vi "SiCenterFinder4Fids.vi"(0 "Operation":enum16{"Manual", "Automatic"}(ring)=enum."Automatic", 1 "Zone":enum16{"ZoneA", "ZoneB", "ZoneC", "ZoneD"}(ring), 2 "Autofocus":T2={"Enable"=TRUE, "InitialStepSize"=0.05, "Tolerance"=0.02, "Abort"=FALSE} {"Tolerance" format="%#_13g"}, 5 "Component":enum16{"Si", "SiOnBP"}(ring), 7 "VisibilityInCamera":enum16{"JoyStick", "AllVisible"}(ring)=enum."AllVisible", 11 "error in (no error)":errorcluster, 12 "Position":enum16{"1", "2"}(ring), 14 "SaveImagesLog":bool) -> (4 "Output XYZU":string, 6 "Image":T4(plugin-control), 8 "Image 2":T4[](array[plugin-control]) caption="AllImages", 15 "error out":errorcluster)   [LabVIEW 2021]
uses:
  <vilib>/userDefined/High Color/IMAQdx.ctl
  <vilib>/Analysis/coordinate.llb/2D Cartesian Coordinate Rotation (Scalar).vi
  <vilib>/Analysis/baseanly.llb/Mean (DBL).vi
  include/GlobalVariables.vi
  <vilib>/Analysis/NI_AALPro.lvlib
  <vilib>/Analysis/NI_AALBase.lvlib
  <vilib>/vision/driver/NI_Vision_Acquisition_Software.lvlib
panel:
  out "JoyStickStatus":bool
  out "Angle12":dbl
  out "Angle34":dbl
  in  "Camera":T1="cam1"
  in  "MatchParameters":T3={"Number of Matches Requested"=1, "Minimum Match Score"=700.0, "Angle Ranges"=[{"Start Angle"=0.0, "End Angle"=0.0}]}
  out "OutputFile":string
  out "spreadsheet string 2":string
  out "spreadsheet string":string
  in  "ModuleName":string="T1"
  out "SyringeY":dbl format="%#_7g"
  out "SyringeX":dbl format="%#_7g"
  in  "CamToSyringeYoffset":dbl=126.651
  in  "CamToSyringeXoffset":dbl=167.702
  out "FileUsedForFiducials":string
  out "UsedCoordinates":string
  out "CameraGcode":string
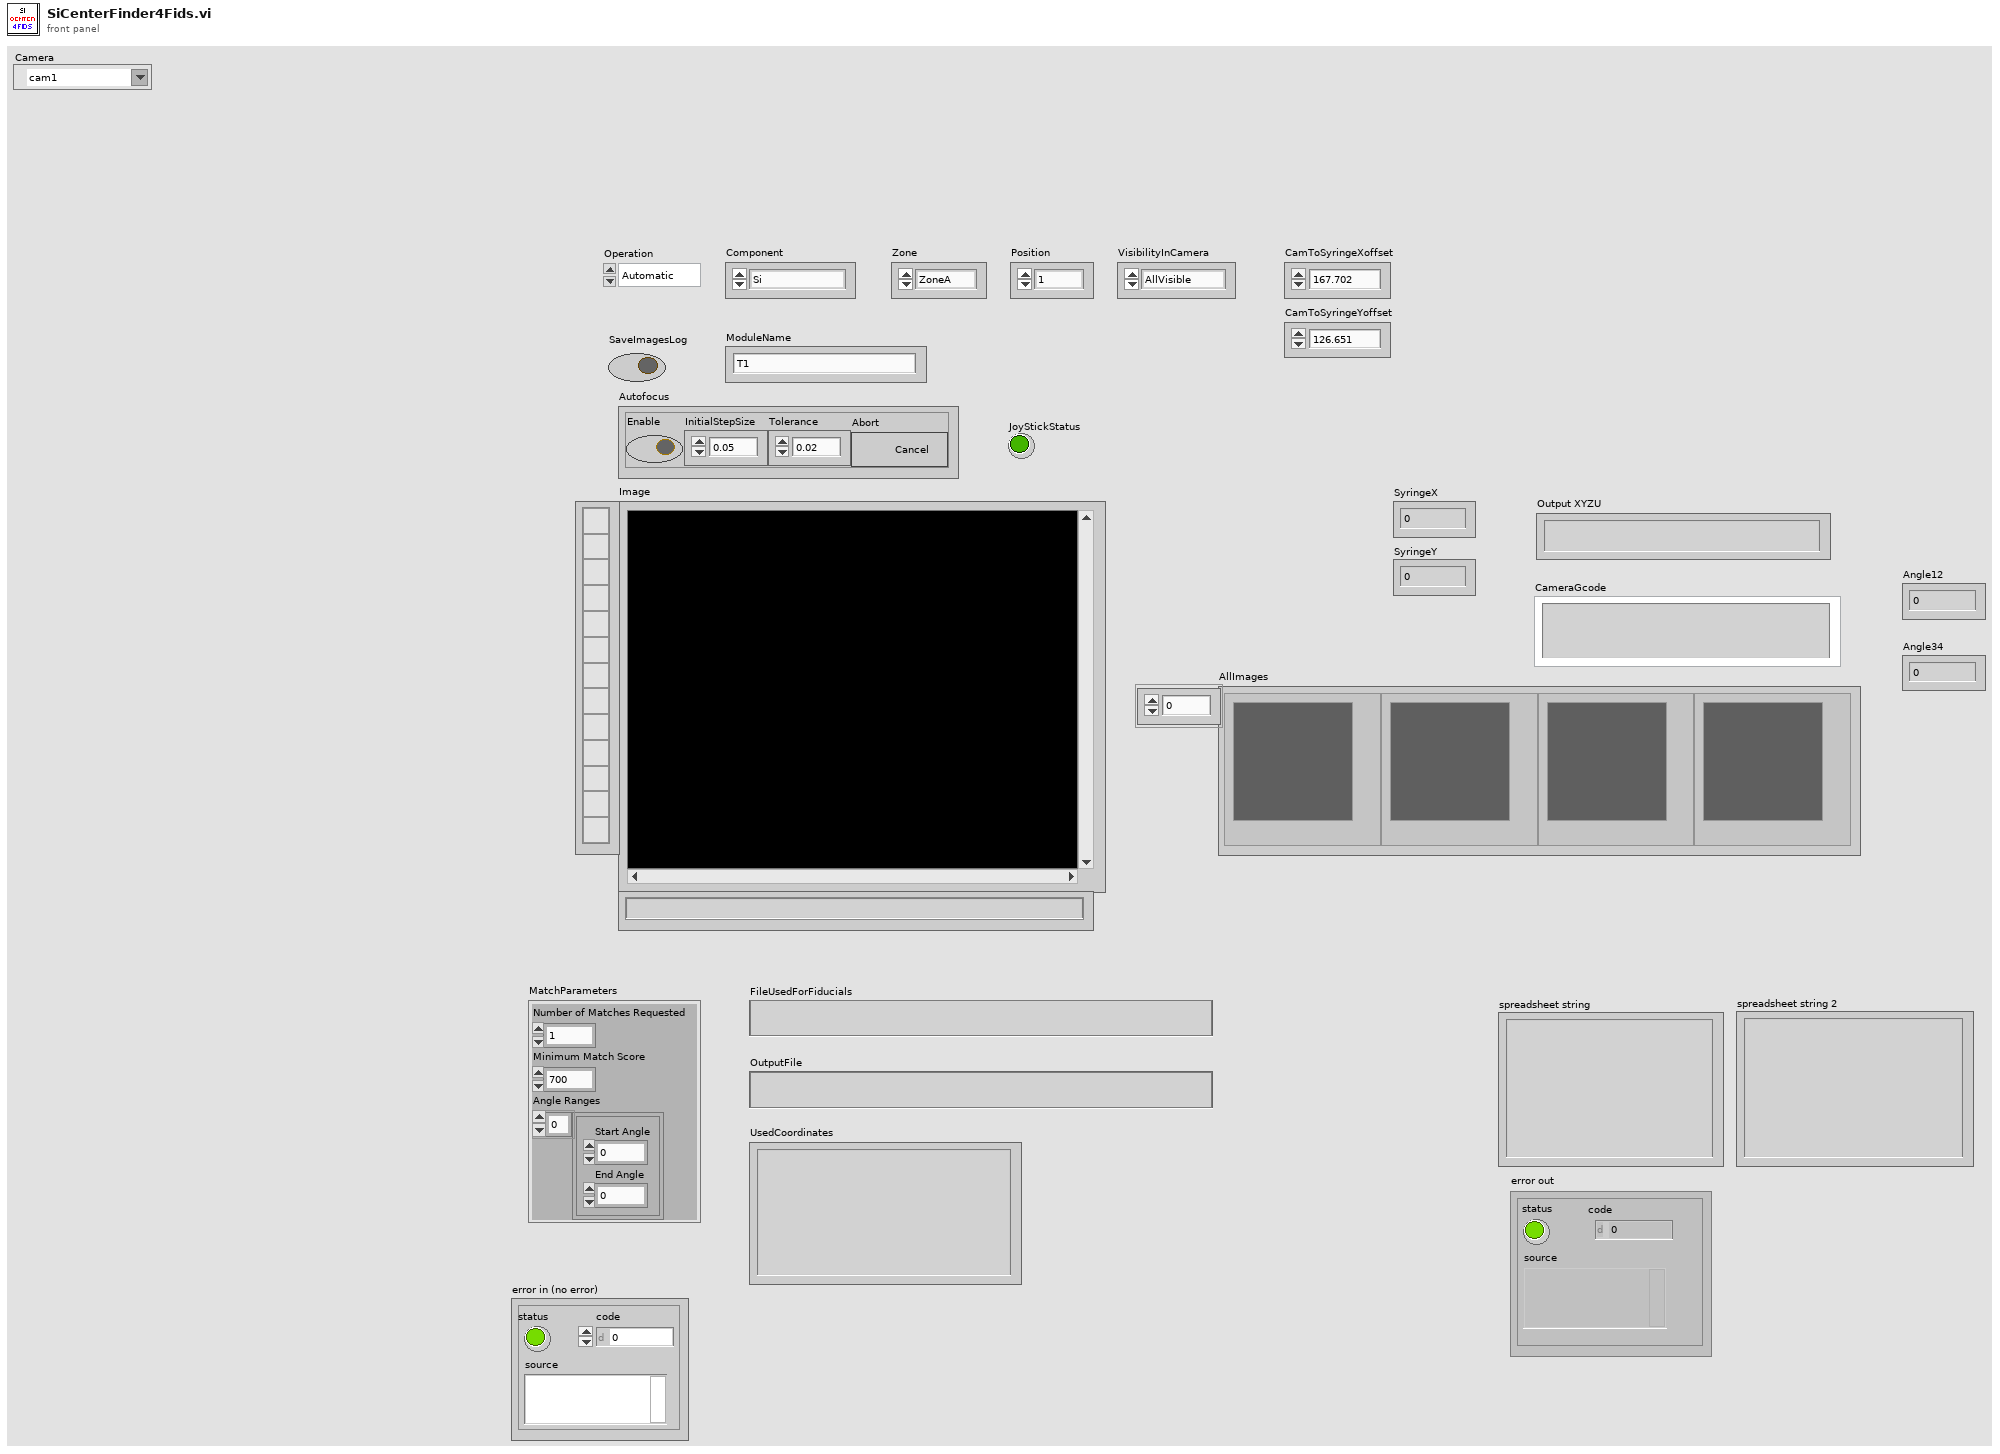
[diagram p1: front panel]
types:
  T1 = typedef "IMAQdx.ctl" = refnum<k21>
  T2 = cluster{"Enable":bool, "InitialStepSize":dbl, "Tolerance":dbl, "Abort":bool}
  T3 = cluster{"Number of Matches Requested":i32, "Minimum Match Score":sgl, "Angle Ranges":cluster{"Start Angle":sgl, "End Angle":sgl}[]}
  T4 = typedef "IMAQ Image.ctl" = refnum<image>
  T5 = typedef "Image Type" = u32
  T6 = typedef "IMAQ Point" = cluster{"X":sgl, "Y":sgl}
  T7 = enum16{"Left Button", "Center Button", "Right Button", "Window Close"}
  T8 = enum16{"open", "replace", "create", "open or create", "replace or create", "replace or create with confirmation"}
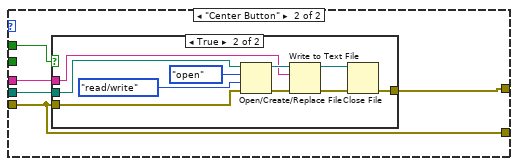
[diagram p5: hidden frame]
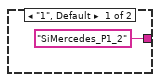
[diagram p7: hidden frame]
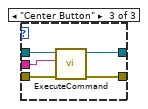
[diagram p10: hidden frame]
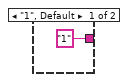
[diagram p11: hidden frame]
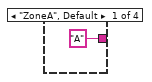
[diagram p12: hidden frame]
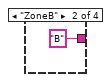
[diagram p13: hidden frame]
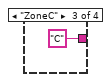
[diagram p14: hidden frame]
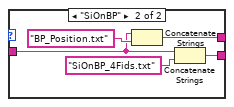
[diagram p15: hidden frame]
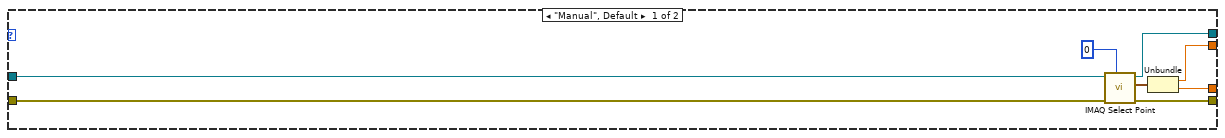
[diagram p16: hidden frame]
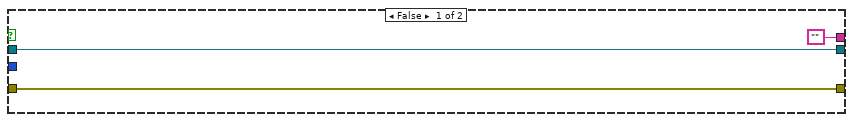
[diagram p18: hidden frame]
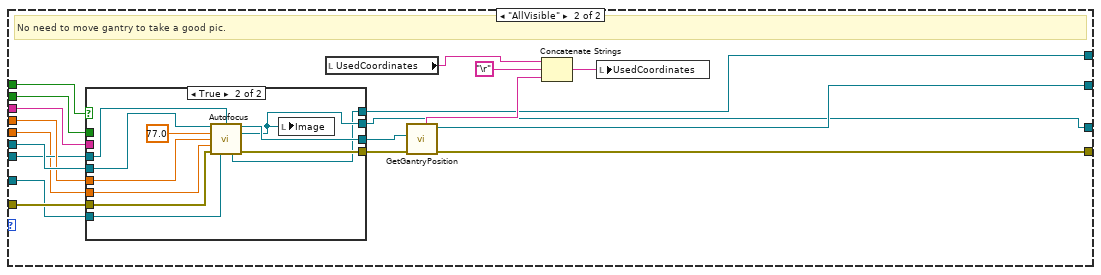
[diagram p20: hidden frame]
diagram:
  w18 = 2 ("y")
  w3 = "Calculated center and current position differ by > 13 um in X or Y or both. Something went wrong with calibration." ("ErrorMessage")
  w5 = "Sensor may not be placed with correct orientation." ("ErrorMessage")
  w33 = -20.0 ("lower limit")
  w32 = 20.0 ("upper limit")
  w55 = ""
  w83 = "%f" ("format string")
  w115 = "\t"
  w112 = i16 6 ("width (-)")
  # "Write the XYZU of the baseplate to a text file & move the gantry?"
  # "Prepare to move the gantry to see the center of component in camera."
  # "AllVisble: Assumes that you know the coordinates of all corners (fiducials) well. No need for any adjustments.\nJoyStick: Use joystick at each point to make good image.\nClickMove: Use \"AdjustCamera\" panel and move the gantry stepwise. Click \"Done\" when you're satisfied with the picture."
  n1 = flat-sequence {
    tunnel: [w126] -> w80
    tunnel: w80 -> [w142]
    tunnel: [w141] -> w79
    tunnel: [w140] -> w77
    tunnel: [w139] -> w74
    tunnel: w79 -> [w179]
    tunnel: [w179] -> w78
    tunnel: w77 -> [w172]
    tunnel: [w169] -> w76
    tunnel: [w178] -> w75
    tunnel: w74 -> [w177]
    tunnel: [w177] -> w73
    tunnel: [w168] -> w65
    tunnel: [w167] -> w64
    tunnel: 4 -> [w206]
    tunnel: [w205] -> w85
    tunnel: [w204] -> w84
    tunnel: [w203] -> w121
    tunnel: [w202] -> w66
    tunnel: [w201] -> w98
    tunnel: "VisibilityInCamera" -> [w200]
    tunnel: [w199] -> w87
    tunnel: w78 -> [w198]
    tunnel: w76 -> [w197]
    tunnel: w75 -> [w196]
    tunnel: w73 -> [w195]
    tunnel: [w195] -> w72
    tunnel: [w194] -> w71
    tunnel: w65 -> [w186]
    tunnel: w64 -> [w188]
    tunnel: [w187] -> w62
    tunnel: [w186] -> w60
    frame #0 {
      n2 = case shown="\"ZoneD\"" "Zone" {
        tunnel: ["A" "B" "C" "D"] -> w130
        frame "ZoneA", Default {
        }
        frame "ZoneB" {
        }
        frame "ZoneC" {
        }
        frame "ZoneD" {
        }
      }
      n3 = case shown="\"2\"" "Position" {
        tunnel: ["1" "2"] -> w131
        frame "1", Default {
        }
        frame "2" {
        }
      }
      n4 = Concatenate Strings(w130, w131, "_" ("string")) -> (w126:string)
      "UsedCoordinates" <- ""
    }
    frame #1 {
      n5 = Concatenate Strings("C:\\Users\\TTUHEP\\Documents\\LabVIEW\\GantryPrograms\\", "Configs\\" ("string"), w142) -> (w149:string)
      n6 = case shown="\"Si\"" "Component" {
        tunnel: w149 -> [w158 w163]
        tunnel: [w160 w165] -> w152
        tunnel: [w157 w162] -> w139
        frame "Si" {
          n7 = Concatenate Strings(w158, "Si_Position.txt") -> (w157:string)
          n8 = Concatenate Strings(w158, "Si_4Fids.txt") -> (w160:string)
        }
        frame "SiOnBP" {
          n9 = Concatenate Strings(w163, "BP_Position.txt") -> (w162:string)
          n10 = Concatenate Strings(w163, "SiOnBP_4Fids.txt") -> (w165:string)
        }
      }
      "FileUsedForFiducials" <- w152
      "OutputFile" <- w139
      n11 = String To Path(string=w152) -> (path=w150:path)
      n12 = Concatenate Strings("This file does not exist:" ("ErrorMessage"), w152) -> (w153:string)
      n13 = call <vilib>:"Check if File or Folder Exists.vi"("error in (no error)"="error in (no error)", "path"=w150) -> ("error out"=w151:errorcluster, "file or folder exists?"=w154:bool, "dup path"=w141:path)  [unwired: 7 in]
      n14 = Not(x=w154) -> (.not. x?=w155:bool)
      n15 = call "AddError.vi"("NoErrorMessage"="InFile OK", "ErrorMessage"=w153, "error in"=w151, "code"=-995, "Error?"=w155) -> ("Error out"=w140:errorcluster)  [unwired: 6 in]
    }
    frame #2 {
      w173 = T5 0 items=["Grayscale (U8)", "Grayscale (I16)", "Grayscale (SGL)", "Complex (CSG)", "RGB (U32)", "HSL (U32)", "RGB (U64)", "Grayscale (U16)"] ("Image Type")
      # "Set the size of the window while selecting the point."
      n16 = call "IMAQ WindSize"("Scrollbars? (N)"=TRUE, "Width & Height"=cluster{"Width":i32, "Height":i32} {"Width"=1333, "Height"=1000}, "Window Number"=0) -> ()  [unwired: 3 in, 3 out]
      n17 = call "IMAQ Create"("Image Name"="name1" ("ImageName"), "Image Type"=w173, "error in (no error)"=w172) -> ("New Image"=w168:T4, "error out"=w175:errorcluster)  [unwired: 2 in]
      n18 = call "Connect.vi"("error in (no error)"=w172) -> ("error out"=w181:errorcluster, "controller"=w182:refnum<k24>)  [unwired: 9 in]
      n19 = call <vilib>:"IMAQdx Open Camera.vi"("error in"=w175, "Session In"="Camera") -> ("error out"=w171:errorcluster, "Session Out"=w167:T1)  [unwired: 8 in]
      n20 = call "ExecuteCommand.vi"("error in (no error)"=w181, "Command Code"="G90\nG1 Z0 F100", "controller in"=w182) -> ("error out"=w170:errorcluster, "controller out"=w178:refnum<k24>)  [unwired: 6 in, 1 out]
      n21 = Merge Errors(w171, w170) -> (w169:errorcluster)
    }
    frame #3 {
      n22 = local read "Autofocus"() -> (w193:T2)
      n23 = Unbundle By Name(w193) -> ("Enable"=w192:bool, "Abort"=w191:bool, "InitialStepSize"=w189:dbl, "Tolerance"=w190:dbl)
      n24 = for {
        N: w206 -> [_]
        tunnel: w197 -> [w249]
        tunnel: w196 -> [w267]
        tunnel: w198 -> [w250]
        tunnel: [w247] -> w205 mode=indexing
        tunnel: [w246] -> w204 mode=indexing
        tunnel: [w245] -> w203 mode=indexing
        tunnel: [w232] -> w202 mode=indexing
        tunnel: [w242] -> w201
        tunnel: w200 -> [w241]
        tunnel: w191 -> [w240]
        tunnel: w192 -> [w239]
        tunnel: w189 -> [w238]
        tunnel: [w234] -> w199
        tunnel: [w229] -> w194 mode=indexing
        tunnel: w190 -> [w217]
        tunnel: w186 -> [w215]
        tunnel: w188 -> [w212]
        tunnel: [w208] -> w187
        i -> [w218]
        w219 = T5 6 items=["Grayscale (U8)", "Grayscale (I16)", "Grayscale (SGL)", "Complex (CSG)", "RGB (U32)", "HSL (U32)", "RGB (U64)", "Grayscale (U16)"] ("Image Type")
        # "Array of XY cluser"
        # "Z array"
        # "Y array"
        # "X array"
        # "Read text file line by line. Each line contains X,Y,Z coordinates for the gantry."
        n25 = call "GetArrayFmTxtFile.vi"("error in"=w249, "LineNo."=w218, "TextFile"=w250) -> ("error out"=w248:errorcluster, "Array"=w274:dbl[])
        n26 = Index Array(array=w274, index=0) -> (element=w269:dbl)
        n27 = Index Array(array=w274, index=1) -> (element=w268:dbl)
        n28 = Index Array(array=w274, index=2) -> (element=w270:dbl)
        n29 = call "Move.vi"("X"=w269, "Absolute"=TRUE, "Y"=w268, "Z"=w270, "SpeedXY (mm/s)"=100.0, "SpeedZ (mm/s)"=100.0, "Move Z first"=FALSE) -> ("Position Gcode"=w266:string)  [unwired: 8 in]
        n30 = call "ExecuteCommand.vi"("error in (no error)"=w248, "Command Code"=w266, "controller in"=w267) -> ("error out"=w211:errorcluster, "controller out"=w265:refnum<k24>)  [unwired: 6 in, 1 out]
        n31 = call <vilib>:"IMAQdx Snap2.vi"("error in"=w211, "Image In"=w215, "Session In"=w212) -> ("error out"=w210:errorcluster, "Image Out"=w214:T4, "Session Out"=w213:T1)  [unwired: 6 in]
        n32 = local write "Image"(w214) -> ()
        n33 = case shown="\"JoyStick\", Default" w241 {
          tunnel: w213 -> [w361 w409]
          tunnel: w265 -> [w377 w423]
          tunnel: w210 -> [w375 w424]
          tunnel: [w357 w411] -> w236
          tunnel: [w364 w417] -> w254
          tunnel: [w365 w415] -> w209
          tunnel: w214 -> [w356 w410]
          tunnel: w240 -> [w368 w421]
          tunnel: w239 -> [w363 w422]
          tunnel: w238 -> [w362 w420]
          tunnel: "name1" ("ImageName") -> [_ w408]
          tunnel: w217 -> [w359 w407]
          tunnel: [w354 w406] -> w208
          frame "JoyStick", Default {
            # "Use joystick to go to a position where camera sees good image."
            n34 = while {
              tunnel: w361 -> [w403]
              tunnel: [w398] -> w358
              tunnel: w377 -> [w405]
              tunnel: [w401] -> w373
              tunnel: [w405] -> w374
              tunnel: w375 -> [w402]
              tunnel: w356 -> [w404]
              tunnel: [w400] -> w355
              stop <- w399 stop-if-true
              n35 = call <vilib>:"IMAQdx Snap2.vi"("error in"=w402, "Image In"=w404, "Session In"=w403) -> ("error out"=w401:errorcluster, "Image Out"=w398:T4, "Session Out"=w400:T1)  [unwired: 6 in]
              n36 = local write "Image"(w398) -> ()
              n37 = global write "GlobalVariables.vi" "Image"(w398) -> ()
              n38 = local read "JoyStickStatus"() -> (w399:bool)
            }
            n39 = call "ExecuteCommand.vi"("error in (no error)"=w375, "Command Code"="JOYSTICK 2D RESET\nJOYSTICK 2D AXISGROUP 1 Y X\nJOYSTICK 2D AXISGROUP 2 Y Z\nJOYSTICK 2D ON", "controller in"=w377) -> ("error out"=w376:errorcluster, "controller out"=w353:refnum<k24>)  [unwired: 6 in, 1 out]
            n40 = call <vilib>:"Clear Errors.vi"("error in (no error)"=w376) -> ()  [unwired: 5 in, 2 out]
            n41 = call "GetGantryPosition.vi"("error in (no error)"=w373, "Controller In"=w374) -> ("error out"=w369:errorcluster, "controller out"=w367:refnum<k24>, "Position_XYZ"=w360:string)  [unwired: 3 in, 4 out]
            n42 = Not A Number/Path/Refnum?(number/path/refnum=w353) -> (NaN/Path/Refnum?=w352:bool)
            n43 = case shown="True" w363 {
              tunnel: w369 -> [w383 w397]
              tunnel: w368 -> [_ _]
              tunnel: w367 -> [w381 w391]
              tunnel: [w382 w395] -> w366
              tunnel: [w383 w394] -> w365
              tunnel: [w381 w393] -> w364
              tunnel: w360 -> [w382 _]
              tunnel: w362 -> [_ w389]
              tunnel: w359 -> [_ w388]
              tunnel: w358 -> [w380 w385]
              tunnel: [w380 w387] -> w357
              tunnel: w355 -> [w379 w386]
              tunnel: [w379 w384] -> w354
              frame False {
              }
              frame True {
                n44 = call "Autofocus.vi"("controller in"=w391, "ImageIn"=w385, "SafeMaxZ"=77.0, "InitialStepSize"=w389, "Tolerance"=w388, "error in (no error)"=w397, "SessionIn"=w386) -> ("controller out"=w396:refnum<k24>, "Image"=w387:T4, "Session Out"=w384:T1, "error out"=w392:errorcluster)  [unwired: 3 in, 2 out]
                n45 = local write "Image"(w387) -> ()
                n46 = call "GetGantryPosition.vi"("error in (no error)"=w392, "Controller In"=w396) -> ("error out"=w394:errorcluster, "controller out"=w393:refnum<k24>, "Position_XYZ"=w395:string)  [unwired: 3 in, 4 out]
              }
            }
            n47 = local write "JoyStickStatus"(w352) -> ()
            n48 = local read "UsedCoordinates"() -> (w371:string)
            n49 = Concatenate Strings(w371, "\r", w366) -> (w372:string)
            n50 = local write "UsedCoordinates"(w372) -> ()
          }
          frame "AllVisible" {
            # "No need to move gantry to take a good pic."
            n51 = case shown="True" w422 {
              tunnel: w421 -> [_ _]
              tunnel: [w428 w433] -> w416
              tunnel: [w427 w439] -> w418
              tunnel: w424 -> [w428 w436]
              tunnel: w423 -> [w427 w438]
              tunnel: w420 -> [_ w435]
              tunnel: [w426 w432] -> w411
              tunnel: w410 -> [w426 w431]
              tunnel: w409 -> [w425 w430]
              tunnel: w408 -> [_ _]
              tunnel: w407 -> [_ w434]
              tunnel: [w425 w429] -> w406
              frame False {
              }
              frame True {
                n52 = call "Autofocus.vi"("controller in"=w438, "ImageIn"=w431, "SafeMaxZ"=77.0, "InitialStepSize"=w435, "Tolerance"=w434, "error in (no error)"=w436, "SessionIn"=w430) -> ("controller out"=w439:refnum<k24>, "Image"=w432:T4, "Session Out"=w429:T1, "error out"=w433:errorcluster)  [unwired: 3 in, 2 out]
                n53 = local write "Image"(w432) -> ()
              }
            }
            n54 = local read "UsedCoordinates"() -> (w413:string)
            n55 = call "GetGantryPosition.vi"("error in (no error)"=w416, "Controller In"=w418) -> ("error out"=w415:errorcluster, "controller out"=w417:refnum<k24>, "Position_XYZ"=w414:string)  [unwired: 3 in, 4 out]
            n56 = Concatenate Strings(w413, "\r", w414) -> (w412:string)
            n57 = local write "UsedCoordinates"(w412) -> ()
          }
        }
        n58 = case shown="\"Automatic\"" "Operation" {
          tunnel: [w283 w314] -> w262
          tunnel: [w282 w313] -> w261
          tunnel: [w281 w293] -> w260
          tunnel: w209 -> [w280 w311]
          tunnel: w236 -> [w279 w315]
          tunnel: [w278 w289] -> w228
          frame "Manual", Default {
            n59 = call "IMAQ Select Point"("Window Number (0...15)"=0, "error in (no error)"=w280, "Image In"=w279) -> ("error out"=w281:errorcluster, "Point"=w284:T6, "Image Out (duplicate)"=w278:T4)  [unwired: 5 in, 1 out]
            n60 = Unbundle(w284) -> ("X"=w283:sgl, "Y"=w282:sgl)
          }
          frame "Automatic" {
            w297 = "SiFid"
            w309 = ""
            n61 = Concatenate Strings("Could not parse/find this template file for pattern recognition:" ("ErrorMessage"), w297) -> (w304:string)
            n62 = call "JSONfileReader.vi"("error in"=w311, "Variant"=w309, "ItemName"=w297, "FileIn"=path "C:/Users/TTUHEP/Documents/LabVIEW/GantryPrograms/Configs/PatternRecognTemplateMaps.json" ("PatterRecognTemplateMap")) -> ("error out"=w301:errorcluster, "Data"=w310:variant, "Found"=w307:bool)
            n63 = Not(x=w307) -> (.not. x?=w306:bool)
            n64 = Variant To Data(error in=w301, type=w309, Variant=w310) -> (data=w308:string, error out=w300:errorcluster)
            n65 = call "AddError.vi"("NoErrorMessage"="Template file name found from json.", "ErrorMessage"=w304, "error in"=w300, "code"=-902, "Error?"=w306) -> ("Error out"=w299:errorcluster)  [unwired: 6 in]
            n66 = call "PatternRecognition.vi"("error in (no error)"=w299, "MatchParameters"="MatchParameters", "ImageIn"=w315, "TemplateFileName"=w308) -> ("error out"=w287:errorcluster, "Position"=w292:cluster{"x":sgl, "y":sgl}, "ImageFoundPattern"=w290:T4, "Number of Matches"=w296:i32)  [unwired: 2 in, 1 out]
            n67 = Equal?(x=w296, y=1) -> (x = y?=w294:bool)
            n68 = call <vilib>:"Clear Errors.vi"("error in (no error)"=w287, "specific error code to clear (0: all)"=-903) -> ("error out"=w286:errorcluster)  [unwired: 4 in, 1 out]
            n69 = case shown="False" w294 {
              tunnel: w286 -> [w320 w324]
              tunnel: [w319 w324] -> w293
              tunnel: w292 -> [_ w323]
              tunnel: [w318 w323] -> w291
              tunnel: w290 -> [w317 w322]
              tunnel: [w316 w322] -> w289
              frame False {
                n70 = call "IMAQ Select Point"("Window Number (0...15)"=0, "error in (no error)"=w320, "Image In"=w317) -> ("error out"=w319:errorcluster, "Point"=w318:T6, "Image Out (duplicate)"=w316:T4)  [unwired: 5 in, 1 out]
              }
              frame True {
              }
            }
            n71 = Unbundle(w291) -> ("X"=w314:sgl, "Y"=w313:sgl)
          }
        }
        n72 = Number To Decimal String(number=w218) -> (decimal integer string=w227:string)  [unwired: 1 in]
        n73 = Concatenate Strings("imgTemp" ("string"), w227) -> (w224:string)
        n74 = call "GetPixelToGantryRelPosition.vi"("error in (no error)"=w260, "PixelY"=w261, "PixelX"=w262) -> ("error out"=w222:errorcluster, "YmmRelGH"=w258:dbl, "XmmRelGH"=w259:dbl)
        n75 = call "IMAQ Create"("Image Name"=w224, "Image Type"=w219, "error in (no error)"=w222) -> ("New Image"=w223:T4, "error out"=w221:errorcluster)  [unwired: 2 in]
        n76 = call "IMAQ Copy"("error in (no error)"=w221, "Image Dst"=w223, "Image Src"=w228) -> ("error out"=w220:errorcluster, "Image Dst Out"=w225:T4)  [unwired: 3 in]
        n77 = Build Array(w225) -> (w229:T4[])
        n78 = flat-sequence {
          tunnel: w220 -> [w343]
          tunnel: [w343] -> w264
          tunnel: w254 -> [w342]
          tunnel: [w342] -> w263
          tunnel: [w351] -> w233
          tunnel: [w350] -> w257
          tunnel: [w349] -> w256
          tunnel: [w348] -> w242
          tunnel: [w347] -> w255
          tunnel: w264 -> [w346]
          tunnel: w263 -> [w345]
          frame #0 {
            n79 = Wait (ms)(milliseconds to wait=u32 1000) -> ()  [unwired: 1 out]
          }
          frame #1 {
            n80 = call "GetGantryPosition.vi"("error in (no error)"=w346, "Controller In"=w345) -> ("error out"=w351:errorcluster, "Position Y"=w350:dbl, "Position X"=w349:dbl, "controller out"=w348:refnum<k24>, "Position Z"=w347:dbl)  [unwired: 3 in, 2 out]
          }
        }
        n81 = Add(x=w259, y=w256) -> (x+y=w253:dbl)
        n82 = Add(x=w258, y=w257) -> (x+y=w252:dbl)
        n83 = case shown="True" "SaveImagesLog" {
          tunnel: w228 -> [w325 w341]
          tunnel: w218 -> [_ w339]
          tunnel: ["" w331] -> w234
          tunnel: w233 -> [w326 w330]
          tunnel: [w326 w329] -> w232
          tunnel: [w325 w328] -> w216
          frame False {
          }
          frame True {
            w333 = "C:\\Users\\TTUHEP\\Documents\\LabVIEW\\GantryPrograms\\LogFiles\\CalibrationData\\"
            n84 = Number To Decimal String(number=w339) -> (decimal integer string=w337:string)  [unwired: 1 in]
            n85 = Concatenate Strings(w333, "ModuleName") -> (w331:string)
            n86 = Concatenate Strings(w333, "ModuleName", "Image" ("string"), w337, ".png" ("string")) -> (w335:string)
            n87 = String To Path(string=w335) -> (path=w334:path)
            n88 = call-poly "IMAQ Write File 2"("error in (no error)"=w330, "Image Quality"=u32 1000, "File Path"=w334, "Image"=w341) -> ("error out"=w329:errorcluster, "Image Out (duplicate)"=w328:T4)  [unwired: 6 in]
          }
        }
        "Image" <- w216
        n89 = call-poly <vilib>:"2D Cartesian Coordinate Rotation.vi"("theta"=0.0, "y"=w252, "x"=w253) -> ("y out"=w243:dbl, "x out"=w244:dbl)  [unwired: 6 in, 1 out]
        n90 = global write "GlobalVariables.vi" "Image"(w216) -> ()
        n91 = Build Array(w255) -> (w245:dbl[])
        n92 = Build Array(w243) -> (w246:dbl[])
        n93 = Build Array(w244) -> (w247:dbl[])
        "JoyStickStatus" <- TRUE ("NaN/Path/Refnum?")
      }
    }
  }
  n94 = Array To Spreadsheet String(array=w84, 3:w83) -> (spreadsheet string=→"spreadsheet string 2":string)  [unwired: 1 in]
  n95 = Array To Spreadsheet String(array=w85, 3:w83) -> (spreadsheet string=→"spreadsheet string":string)  [unwired: 1 in]
  n96 = String To Path(string=w72) -> (path=w38:path)
  n97 = Index Array(array=w71, index (col)=0 ("disabled index (col)")) -> (element=→"Image 2":T4[])  [unwired: 1 in]
  n98 = Index Array "Y"(array=w84, index (col)=0 ("disabled index (col)")) -> (element=w118:dbl[])  [unwired: 1 in]
  n99 = Index Array "X"(array=w85, index (col)=0 ("disabled index (col)")) -> (element=w119:dbl[])  [unwired: 1 in]
  n100 = Index Array "Z"(array=w121, index (col)=0 ("disabled index (col)")) -> (element=w120:dbl[])  [unwired: 1 in]
  n101 = formula code="float64 m1 = 0.0, m2 = 0.0, x = 0.0, y = 0.0;\nfloat64 orientn = 0.0, angl1 = 0.0, angl2 = 0.0;\n\nm1 = (yin[1] - yin[0]) / (xin[1] - xin[0]);\nm2 = (yin[2] - yin[3]) / (xin[2] - xin[3]);\nangl1 = (atan(m1)*180.0/3.14159);\nangl2 = (atan(m2)*180.0/3.14159);\norientn = 0.5*(angl1+angl2);\n\nx = 0.25*(xin[0]+xin[1]+xin[2]+xin[3]);\ny = 0.25*(yin[0]+yin[1]+yin[2]+yin[3]);"("xin"=w119, "yin"=w118) -> ("orientn"=w99:dbl, "x"=w68:dbl, "y"=w67:dbl, "angl1"=→"Angle34" →"Angle12":dbl)  [unwired: 1 out]
  n102 = call-poly <vilib>:"Mean.vi"("X"=w120) -> ("mean"=w100:dbl)  [unwired: 1 out]
  n103 = Number To Fractional String(number=w68, precision (6)=w112) -> (F-format string=w117:string)  [unwired: 2 in]
  n104 = Number To Fractional String(number=w67, precision (6)=w112) -> (F-format string=w116:string)  [unwired: 2 in]
  n105 = Number To Fractional String(number=w100, precision (6)=w112) -> (F-format string=w111:string)  [unwired: 2 in]
  n106 = call "CameraXYusingGantryHeadXY.vi"("GantryY"=w67, "GantryX"=w68) -> ("CamY"=w91:dbl, "CamX"=w93:dbl)
  n107 = Number To Fractional String(number=w99, precision (6)=i16 4 ("width (-)")) -> (F-format string=w113:string)  [unwired: 2 in]
  n108 = call "Move.vi"("X"=w93, "Absolute"=TRUE, "Y"=w91, "Z"=w100, "SpeedXY (mm/s)"=100.0, "SpeedZ (mm/s)"=50.0, "Move Z first"=TRUE) -> ("Position Gcode"=w102:string)  [unwired: 8 in]
  "CameraGcode" <- w102
  n109 = Add(x="CamToSyringeYoffset", y=w91) -> (x+y=→"SyringeY":dbl)
  n110 = Concatenate Strings(w117, w115, w116, w115, w111, w115, w113, "\r") -> (w37:string)
  "Output XYZU" <- w37
  n111 = Add(x="CamToSyringeXoffset", y=w93) -> (x+y=→"SyringeX":dbl)
  n112 = Concatenate Strings("Overwrite/Append ", w37, " to file ", w72, " ?" ("string")) -> (w107:string)
  n113 = call <vilib>:"Three Button Dialog.vi"("Right Button Text (\"Cancel\")"="Do nothing" ("Right Button Text (\"Cancel\")"), "Center Button Text (\"No\")"="Append" ("Center Button Text (\"No\")"), "Left Button Text (\"Yes\")"="Overwrite" ("Left Button Text (\"Yes\")"), "message"=w107) -> ("Which Button?"=w41:T7)  [unwired: 7 in]
  n114 = Merge Errors(w66) -> (w63:errorcluster)
  n115 = case shown="\"Left Button\", Default" w41 {
    tunnel: w63 -> [w444 w446 w451]
    tunnel: w102 -> [w443 _ w450]
    tunnel: w98 -> [w442 w445 w449]
    tunnel: [w440 w446 w447] -> w61
    tunnel: [w441 w445 w448] -> w101
    frame "Left Button", Default {
      n116 = call "ExecuteCommand.vi"("error in (no error)"=w444, "Command Code"=w443, "controller in"=w442) -> ("error out"=w440:errorcluster, "controller out"=w441:refnum<k24>)  [unwired: 6 in, 1 out]
    }
    frame "Right Button" {
    }
    frame "Center Button" {
      n117 = call "ExecuteCommand.vi"("error in (no error)"=w451, "Command Code"=w450, "controller in"=w449) -> ("error out"=w447:errorcluster, "controller out"=w448:refnum<k24>)  [unwired: 6 in, 1 out]
    }
  }
  n118 = local read "Position"() -> (w43:enum16{"1", "2"})
  n119 = case shown="\"2\"" w43 {
    tunnel: ["SiMercedes_P1_2" "SiMercedes_P2_2"] -> w42
    frame "1", Default {
    }
    frame "2" {
    }
  }
  n120 = call <vilib>:"IMAQdx Snap2.vi"("error in"=w61, "Image In"=w60, "Session In"=w62) -> ("error out"=w58:errorcluster, "Image Out"=w22:T4, "Session Out"=w59:T1)  [unwired: 6 in]
  n121 = local write "Image"(w22) -> ()
  n122 = global write "GlobalVariables.vi" "Image"(w22) -> ()
  n123 = call <vilib>:"IMAQdx Close Camera.vi"("error in"=w58, "Session In"=w59) -> ("error out"=w25:errorcluster)  [unwired: 9 in]
  n124 = call "Disconnect.vi"("error in (no error)"=w25, "controller"=w101) -> ("error out"=w24:errorcluster)  [unwired: 9 in]
  n125 = Concatenate Strings("Could not parse/find this template file for pattern recognition:" ("ErrorMessage"), w42) -> (w50:string)
  n126 = call "JSONfileReader.vi"("error in"=w24, "Variant"=w55, "ItemName"=w42, "FileIn"=path "C:/Users/TTUHEP/Documents/LabVIEW/GantryPrograms/Configs/PatternRecognTemplateMaps.json" ("PatterRecognTemplateMap")) -> ("error out"=w47:errorcluster, "Data"=w56:variant, "Found"=w53:bool)
  n127 = Not(x=w53) -> (.not. x?=w52:bool)
  n128 = Variant To Data(error in=w47, type=w55, Variant=w56) -> (data=w54:string, error out=w46:errorcluster)
  n129 = call "AddError.vi"("NoErrorMessage"="Template file name found from json.", "ErrorMessage"=w50, "error in"=w46, "code"=-902, "Error?"=w52) -> ("Error out"=w45:errorcluster)  [unwired: 6 in]
  n130 = local read "MatchParameters"() -> (w44:T3)
  n131 = call "PatternRecognition.vi"("error in (no error)"=w45, "MatchParameters"=w44, "ImageIn"=w22, "TemplateFileName"=w54) -> ("error out"=w21:errorcluster, "Position"=w34:cluster{"x":sgl, "y":sgl}, "ImageFoundPattern"=w7:T4, "Number of Matches"=w36:i32)  [unwired: 2 in, 1 out]
  n132 = local write "Image"(w7) -> ()
  n133 = Unbundle(w34) -> ("x"=w16:sgl, "y"=w15:sgl)
  n134 = call "IMAQ GetImageSize"("Image"=w22, "error in (no error)"=w21) -> ("Y Resolution"=w19:i32, "X Resolution"=w20:i32, "error out"=w11:errorcluster)  [unwired: 2 in]
  n135 = Equal?(x=w36, y=1) -> (x = y?=w31:bool)
  n136 = Divide(x=w20, y=w18) -> (x/y=w17:dbl)
  n137 = Divide(x=w19, y=w18) -> (x/y=w14:dbl)
  n138 = Not(x=w31) -> (.not. x?=w6:bool)
  n139 = Subtract(x=w17, y=w16) -> (x-y=w13:dbl)
  n140 = Subtract(x=w14, y=w15) -> (x-y=w12:dbl)
  n141 = case shown="True" w6 {
    tunnel: w5 -> [_ w454]
    frame False {
    }
    frame True {
      n142 = One Button Dialog(message=w454) -> ()  [unwired: 1 in, 1 out]
    }
  }
  n143 = In Range and Coerce(upper limit=w32, x=w13, lower limit=w33) -> (In Range?=w29:bool)  [unwired: 1 out]
  n144 = In Range and Coerce(upper limit=w32, x=w12, lower limit=w33) -> (In Range?=w28:bool)  [unwired: 1 out]
  n145 = call "AddError.vi"("NoErrorMessage"="Sensor orientation is OK.", "ErrorMessage"=w5, "error in"=w11, "code"=-912, "Error?"=w6) -> ("Error out"=w4:errorcluster)  [unwired: 6 in]
  n146 = Compound Arithmetic op=AND(w31, w29, w28) -> (w26:bool)
  n147 = Compound Arithmetic op=AND(w29, w28) -> (w27:bool)
  n148 = Not(x=w27) -> (.not. x?=w2:bool)
  n149 = case shown="True" w2 {
    tunnel: w3 -> [_ w455]
    frame False {
    }
    frame True {
      n150 = One Button Dialog(message=w455) -> ()  [unwired: 1 in, 1 out]
    }
  }
  n151 = call "AddError.vi"("ErrorMessage"=w3, "error in"=w4, "code"=-913, "Error?"=w2) -> ("Error out"=w8:errorcluster)  [unwired: 7 in]
  n152 = case shown="\"Left Button\", Default" w41 {
    tunnel: w38 -> [w460 w479]
    tunnel: w37 -> [w459 w480]
    tunnel: [w456 w476] -> _
    tunnel: w26 -> [_ w478]
    tunnel: w26 -> [w458 _]
    tunnel: [w457 w477] -> w23
    tunnel: w8 -> [w456 w476]
    frame "Left Button", Default {
      n153 = case shown="True" w458 {
        tunnel: w460 -> [_ w465]
        tunnel: w459 -> [_ w464]
        tunnel: w456 -> [w461 w463]
        tunnel: [w461 w462] -> w457
        frame False {
        }
        frame True {
          n154 = Open/Create/Replace File(file path (use dialog)=w465, error in=w463, operation (0:open)=T8."replace or create", access (0:read/write)=enum16{"read/write", "read-only", "write-only"}."read/write") -> (refnum out=w469:refnum<file>, error out=w467:errorcluster)  [unwired: 2 in, 1 out]
          n155 = Set File Position(offset (in bytes) (0)=i64 0, refnum=w469, from (0:start)=enum16{"start", "end", "current"}."end", error in=w467) -> (refnum out=w468:refnum<file>, error out=w466:errorcluster)
          n156 = Write to Text File(file (use dialog)=w468, text=w464, error in=w466) -> (refnum out=w472:refnum<file>, error out=w473:errorcluster)  [unwired: 1 in, 1 out]
          n157 = Close File(refnum=w472, error in=w473) -> (error out=w462:errorcluster)  [unwired: 1 out]
        }
      }
    }
    frame "Center Button" {
      n158 = case shown="True" w478 {
        tunnel: w480 -> [_ w485]
        tunnel: w476 -> [w481 w484]
        tunnel: w479 -> [_ w483]
        tunnel: [w481 w482] -> w477
        frame False {
        }
        frame True {
          n159 = Open/Create/Replace File(file path (use dialog)=w483, error in=w484, operation (0:open)=T8."open", access (0:read/write)=enum16{"read/write", "read-only", "write-only"}."read/write") -> (refnum out=w491:refnum<file>, error out=w488:errorcluster)  [unwired: 2 in, 1 out]
          n160 = Write to Text File(file (use dialog)=w491, text=w485, error in=w488) -> (refnum out=w486:refnum<file>, error out=w487:errorcluster)  [unwired: 1 in, 1 out]
          n161 = Close File(refnum=w486, error in=w487) -> (error out=w482:errorcluster)  [unwired: 1 out]
        }
      }
    }
  }
  n162 = local read "SaveImagesLog"() -> (w88:bool)
  n163 = case shown="True" w88 {
    tunnel: w23 -> [w492 w507]
    tunnel: w87 -> [_ w500]
    tunnel: w22 -> [_ w495]
    tunnel: [w492 w493] -> w86
    frame False {
    }
    frame True {
      n164 = Concatenate Strings(w500, "UsedXYZ.txt") -> (w505:string)
      n165 = local read "UsedCoordinates"() -> (w502:string)
      n166 = Concatenate Strings(w500, "CenterImage.png") -> (w498:string)
      n167 = String To Path(string=w505) -> (path=w504:path)
      n168 = String To Path(string=w498) -> (path=w496:path)
      n169 = Open/Create/Replace File(file path (use dialog)=w504, error in=w507, operation (0:open)=T8."open or create", access (0:read/write)=enum16{"read/write", "read-only", "write-only"}."read/write") -> (refnum out=w503:refnum<file>, error out=w511:errorcluster)  [unwired: 2 in, 1 out]
      n170 = Write to Text File(file (use dialog)=w503, text=w502, error in=w511) -> (refnum out=w501:refnum<file>, error out=w510:errorcluster)  [unwired: 1 in, 1 out]
      n171 = Close File(refnum=w501, error in=w510) -> (error out=w494:errorcluster)  [unwired: 1 out]
      n172 = call-poly "IMAQ Write File 2"("error in (no error)"=w494, "Image Quality"=u32 1000, "File Path"=w496, "Image"=w495) -> ("error out"=w493:errorcluster)  [unwired: 6 in, 1 out]
    }
  }
  "error out" <- w86
